vi "Close Document.vi"(0 "object in":refnum<class "Spreadsheet.lvclass">, 5 "error in (no error)":errorcluster) -> (14 "object out":refnum<class "Spreadsheet.lvclass">, 19 "error out":errorcluster)   [LabVIEW 2014, in "Spreadsheet.lvclass"]
uses:
  Spreadsheet.lvclass
  Spreadsheet.lvclass/Spreadsheet.ctl
  Document_class/Document.lvclass
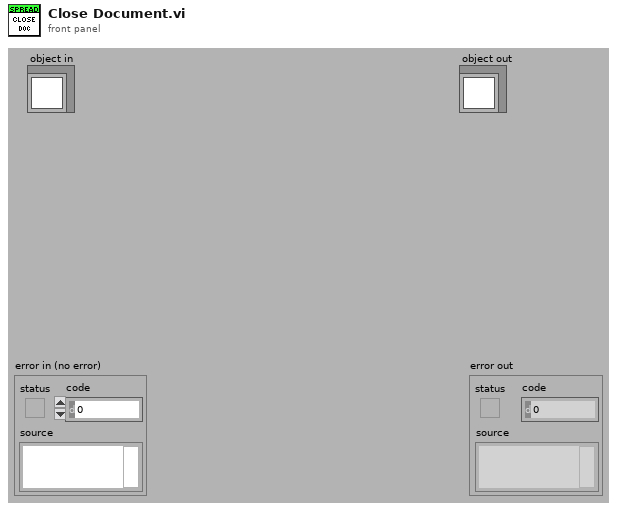
[diagram p1: front panel]
types:
  T1 = cluster{"Table Data":string[][], "Cell Info":string[][], "SheetName":string}[]
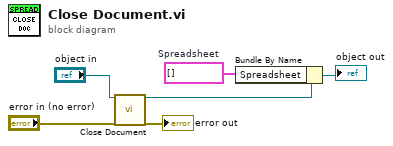
[diagram p0: block diagram]
diagram:
  w2 = T1 []  # Spreadsheet
  n1 = call-parent "Close Document.vi"("object in"="object in", "error in (no error)"="error in (no error)") -> ("object out"=w3:refnum<class "Spreadsheet.lvclass">, "error out"=→"error out":errorcluster)  [unwired: 16 in]
  n2 = Bundle By Name(cluster=w3, "Spreadsheet"=w2) -> (→"object out":refnum<class "Spreadsheet.lvclass">)
